vi "Is 24-bit task.vi"(0 "task":refnum<k21>, 11 "error in (no error)":errorcluster) -> (4 "task out":refnum<k21>, 6 "Product Type":string, 8 "is 24bit?":bool, 10 "PXI?":bool, 14 "Product Category":i32, 15 "error out":errorcluster)   [LabVIEW 2020]
uses:
  <resource>/objmgr/daqmx.rc
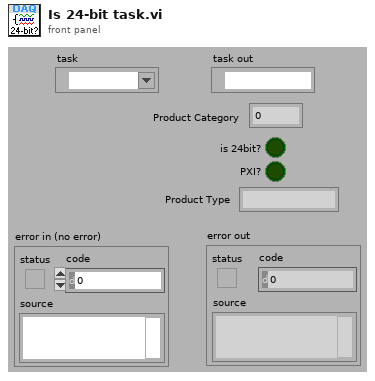
[diagram p1: front panel]
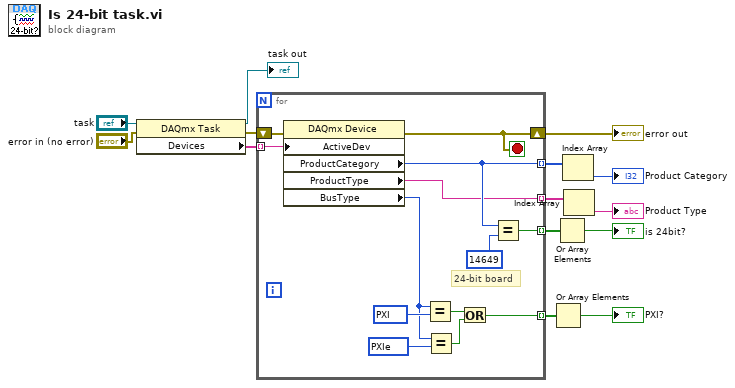
[diagram p0: block diagram]
diagram:
  n1 = property class="DAQmx Task"(reference="task", error in="error in (no error)") -> (reference out=→"task out":refnum<k21>, error out=w12:errorcluster, "Devices"=w13:tag[])
  n2 = for {
    tunnel: w13 -> [w27] mode=indexing
    tunnel: [w24] -> w10 mode=indexing
    tunnel: [w23] -> w6 mode=indexing
    shift-right: [w22] -> w11
    shift-left: w12 -> [w25]
    tunnel: [w19] -> w4 mode=indexing
    tunnel: [w15] -> w2 mode=indexing
    stop <- w22 stop-if-true
    w18 = 14706 items=["PCI"=12582, "PCIe"=13612, "PXI"=12583, "PXIe"=14706, "SCXI"=12584, "SCC"=14707, "PCCard"=12585, "USB"=12586, "CompactDAQ"=14637, "TCP/IP"=14828, "Unknown"=12588, "SwitchBlock"=15870] ("BusType")
    w21 = 12583 items=["PCI"=12582, "PCIe"=13612, "PXI"=12583, "PXIe"=14706, "SCXI"=12584, "SCC"=14707, "PCCard"=12585, "USB"=12586, "CompactDAQ"=14637, "TCP/IP"=14828, "Unknown"=12588, "SwitchBlock"=15870] ("BusType")
    # "24-bit board"
    n3 = property class="DAQmx Device"(error in=w25, "ActiveDev"=w27) -> (error out=w22:errorcluster, "ProductCategory"=w23:i32, "ProductType"=w15:string, "BusType"=w17:i32)  [unwired: 1 in, 1 out]
    n4 = Equal?(x=w17, y=w21) -> (x = y?=w20:bool)
    n5 = Equal?(x=w17, y=w18) -> (x = y?=w16:bool)
    n6 = Or(x=w20, y=w16) -> (x .or. y?=w19:bool)
    n7 = Equal?(x=w23, y=14649) -> (x = y?=w24:bool)
  }
  "error out" <- w11
  n8 = Or Array Elements(Boolean array=w4) -> (logical OR=→"PXI?":bool)
  n9 = Or Array Elements(Boolean array=w10) -> (logical OR=→"is 24bit?":bool)
  n10 = Index Array(array=w6) -> (element=→"Product Category":i32)  [unwired: 1 in]
  n11 = Index Array(array=w2) -> (element=→"Product Type":string)  [unwired: 1 in]
